vi "Pol Data Disp.vi"(5 "poldisplay":dbl[](array[numeric])) -> (1 "poldisp":string[](array[string]))   [LabVIEW 2009]
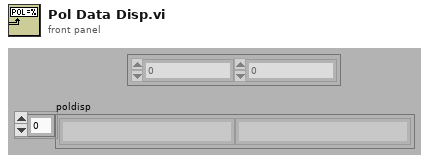
[diagram p1: front panel]
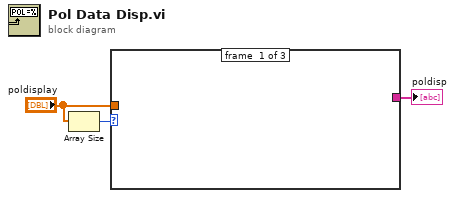
[diagram p0: block diagram]
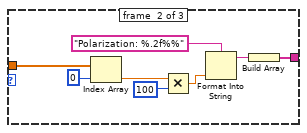
[diagram p2: hidden frame]
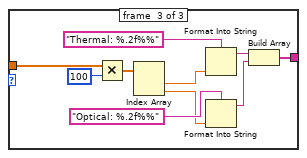
[diagram p3: hidden frame]
diagram:
  n1 = Array Size(array="poldisplay") -> (size(s)=w3:i32)
  n2 = case shown="1" w3 {
    tunnel: [_ w5 w14] -> w2
    tunnel: "poldisplay" -> [_ w11 w19]
    frame #0 {
    }
    frame #1 {
      n3 = Index Array(array=w11, index=0) -> (element=w9:dbl)
      n4 = Multiply(x=w9, y=100) -> (x*y=w7:dbl)
      n5 = Format Into String(format string="Polarization: %.2f%%", w7) -> (resulting string=w4:string)  [unwired: 2 in, 1 out]
      n6 = Build Array(w4) -> (w5:string[])
    }
    frame #2 {
      n7 = Multiply(x=w19, y=100) -> (x*y=w18:dbl[])
      n8 = Index Array(array=w18) -> (element #1=w17:dbl, element #2=w15:dbl)  [unwired: 2 in]
      n9 = Format Into String(format string="Thermal: %.2f%%", w17) -> (resulting string=w13:string)  [unwired: 2 in, 1 out]
      n10 = Format Into String(format string="Optical: %.2f%%", w15) -> (resulting string=w12:string)  [unwired: 2 in, 1 out]
      n11 = Build Array(w13, w12) -> (w14:string[])
    }
  }
  "poldisp" <- w2
